vi "Main.vi"() -> ()   [LabVIEW 2019]
panel:
  out "The winner is:":string
  out "The computer chose:":string
  out "You chose:":string
  in  "Combo Box":string(combo)
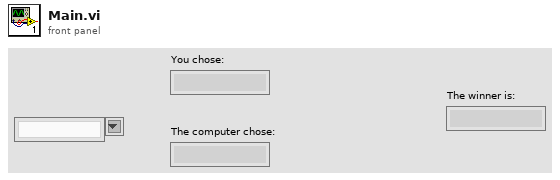
[diagram p1: front panel]
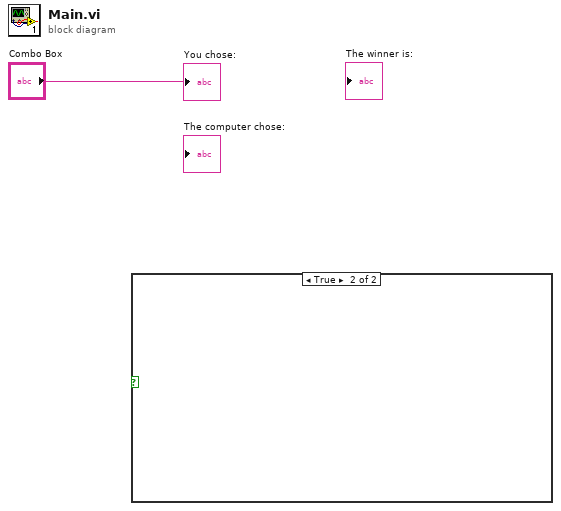
[diagram p0: block diagram]
diagram:
  n1 = case shown="True" {
    selector: _ -> [_ _]
    frame False {
    }
    frame True {
    }
  }
  "You chose:" <- "Combo Box"
